vi "Delete.vi"(8 "error in (no error)":errorcluster, 11 "Child Class in":refnum<class "Instrument.lvclass">) -> (0 "error out":errorcluster, 3 "Child Class out":refnum<class "Instrument.lvclass">)   [LabVIEW 2017, in "Instrument.lvlib" / "Instrument.lvclass"]
uses:
  Instrument.lvclass
  Instrument.lvclass/Instrument.ctl
  Properties/Instrument Properties.lvclass
  <vilib>/TSS/ACRObat Test Framework/Classes/Base Objects/Acrobat Base Object/Acrobat Base Object/Acrobat Base Object.lvclass
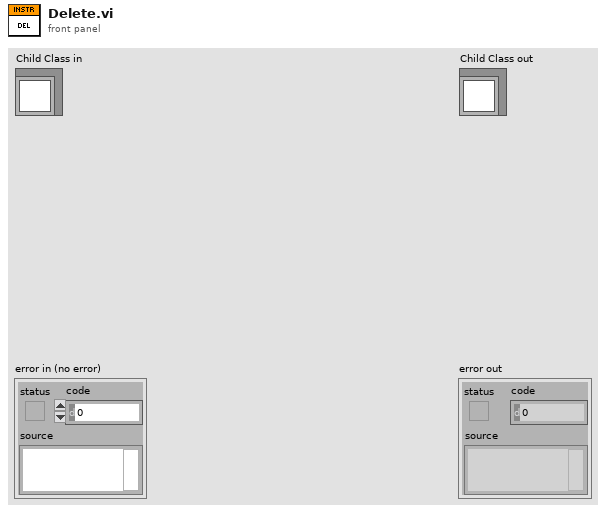
[diagram p1: front panel]
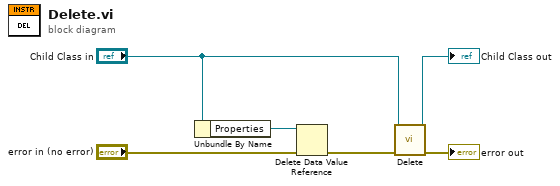
[diagram p0: block diagram]
diagram:
  n1 = Unbundle By Name("Child Class in") -> ("Properties"=w1:refnum<data-value>)
  n2 = Delete Data Value Reference(data value reference=w1, error in="error in (no error)") -> (error out=w2:errorcluster)  [unwired: 1 out]
  n3 = call-parent "Delete.vi"("error in (no error)"=w2, "Child Class in"="Child Class in") -> ("error out"=→"error out":errorcluster, "Child Class out"=→"Child Class out":refnum<class "Instrument.lvclass">)  [unwired: 8 in]
